vi "Splitter.vi"(6 "Selection Colors":T1={"Normal"=13816530, "Mouse-over"=0, "Selected"=9868950, "Selected Mouse-over"=9868950}, 7 "Settings UI Enqueuer":refnum<class "Message Enqueuer.lvclass">, 8 "Error In":errorcluster, 9 "Offset":T2, 10 "Scale Factor":dbl, 11 "Splitter Ref":refnum<vi>) -> (0 "Error Out":errorcluster, 3 "Splitter out":refnum<class "Splitter.lvclass">)   [LabVIEW 2017, in "Splitter.lvclass"]
uses:
  Splitter.lvclass
  D:/software/LabView_PaneRelief_2017/test/D/software/LabView_PaneRelief_2017/Classes/Panel Object/Panel Object.lvclass
  Typedefs/Point--Cluster.ctl
  <vilib>/ActorFramework/Message Enqueuer/Message Enqueuer.lvclass
  Typedefs/Selection Colors--Cluster.ctl
  Typedefs/Splitter Orientation--Enum.ctl
  Splitter.lvclass/Splitter.ctl
  Typedefs/Rectangle--Cluster.ctl
  Panel Object/Panel Object.lvclass/Panel Object.ctl
  Panel Object/Write Bounds.vi
  Panel Object/Write Settings UI Enqueuer.vi
  Panel Object/Write Selection Colors.vi
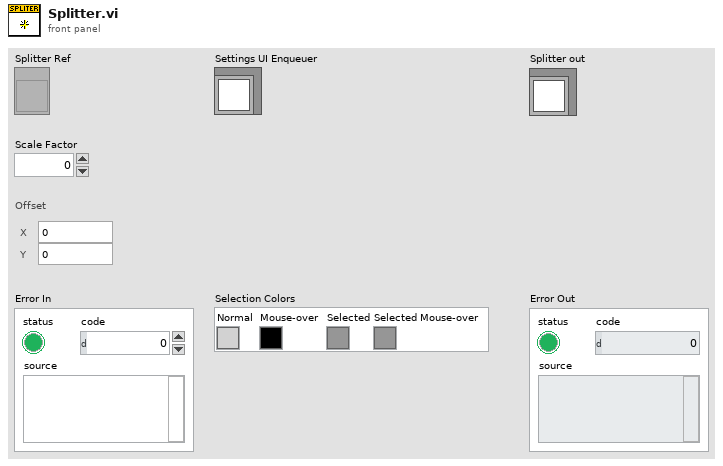
[diagram p1: front panel]
types:
  T1 = typedef "Selection Colors--Cluster.ctl" = cluster{"Normal":u32, "Mouse-over":u32, "Selected":u32, "Selected Mouse-over":u32}
  T2 = typedef "Point--Cluster.ctl" = cluster{"Horizontal":i32, "Vertical":i32}
  T3 = typedef "Splitter Orientation--Enum.ctl" = enum16{"Vertical", "Horizontal"}
  T4 = typedef "Rectangle--Cluster.ctl" = cluster{"X start":i32, "X end":i32, "Y start":i32, "Y end":i32}
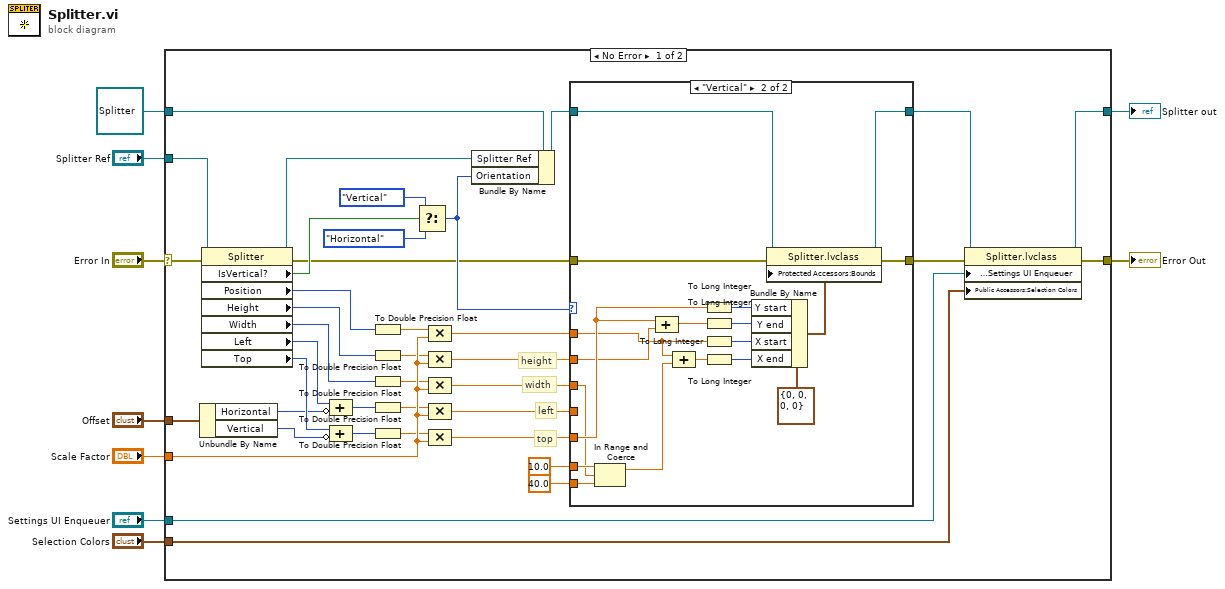
[diagram p0: block diagram]
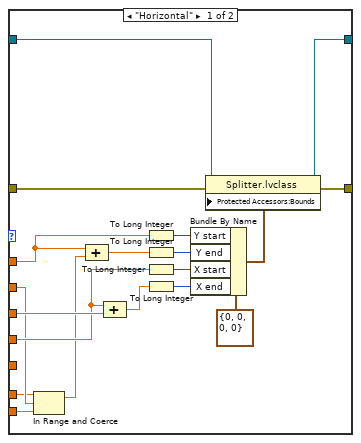
[diagram p2: hidden frame]
diagram:
  n1 = case shown="No Error" "Error In" {
    selector: "Error In" -> [w28 w88]
    tunnel: [w16 w88] -> w7
    tunnel: [w14 w87] -> w9
    tunnel: refnum<class "Splitter.lvclass"> refnum ("Splitter in") -> [w20 w87]
    tunnel: "Splitter Ref" -> [w26 _]
    tunnel: "Scale Factor" -> [w34 _]
    tunnel: "Offset" -> [w33 _]
    tunnel: "Settings UI Enqueuer" -> [w13 _]
    tunnel: "Selection Colors" -> [w12 _]
    frame No Error {
      # "top"
      # "left"
      # "width"
      # "height"
      n2 = Unbundle By Name(w33) -> ("Horizontal"=w35:i32, "Vertical"=w38:i32)
      n3 = property class="Splitter"(reference=w26, error in=w28) -> (reference out=w27:refnum<vi>, error out=w19:errorcluster, "IsVertical?"=w32:bool, "Position"=w48:i32, "Height"=w41:u32, "Width"=w44:u32, "Left"=w37:i32, "Top"=w39:i32)
      n4 = Compound Arithmetic op=ADD(w37, invert w35) -> (w36:i32)
      n5 = Compound Arithmetic op=ADD(w39, invert w38) -> (w40:i32)
      n6 = To Double Precision Float(number=w48) -> (double precision float=w25:dbl)
      n7 = To Double Precision Float(number=w41) -> (double precision float=w24:dbl)
      n8 = To Double Precision Float(number=w44) -> (double precision float=w23:dbl)
      n9 = To Double Precision Float(number=w36) -> (double precision float=w22:dbl)
      n10 = To Double Precision Float(number=w40) -> (double precision float=w21:dbl)
      n11 = Select(t=Splitter_Orientation--Enum."Vertical" ("Splitter Orientation"), s=w32, f=Splitter_Orientation--Enum."Horizontal" ("Splitter Orientation")) -> (s? t:f=w29:T3)
      n12 = Compound Arithmetic op=MULTIPLY(w25, w34) -> (w45:dbl)
      n13 = Compound Arithmetic op=MULTIPLY(w24, w34) -> (w46:dbl)
      n14 = Compound Arithmetic op=MULTIPLY(w23, w34) -> (w47:dbl)
      n15 = Compound Arithmetic op=MULTIPLY(w22, w34) -> (w43:dbl)
      n16 = Compound Arithmetic op=MULTIPLY(w21, w34) -> (w42:dbl)
      n17 = Bundle By Name(cluster=w20, "Splitter Ref"=w27, "Orientation"=w29) -> (w18:refnum<class "Splitter.lvclass">)
      n18 = case shown="\"Vertical\"" w29 {
        tunnel: w45 -> [w64 w83]
        tunnel: w43 -> [w66 _]
        tunnel: w46 -> [w52 w84]
        tunnel: w47 -> [w67 w70]
        tunnel: w42 -> [_ w85]
        tunnel: w19 -> [w58 w77]
        tunnel: [w57 w76] -> w17
        tunnel: [w56 w73] -> w15
        tunnel: w18 -> [w55 w74]
        tunnel: 10.0 ("upper limit") -> [w50 w72]
        tunnel: 40.0 ("upper limit") -> [w49 w71]
        frame "Horizontal" {
          # "Horizontal"
          n19 = In Range and Coerce(upper limit=w50, x=w52, lower limit=w49) -> (coerced(x)=w51:dbl)  [unwired: 1 out]
          n20 = Compound Arithmetic op=ADD(w64, w51) -> (w63:dbl)
          n21 = Compound Arithmetic op=ADD(w66, w67) -> (w65:dbl)
          n22 = To Long Integer(number=w64) -> (32bit integer=w62:i32)
          n23 = To Long Integer(number=w63) -> (32bit integer=w61:i32)
          n24 = To Long Integer(number=w66) -> (32bit integer=w60:i32)
          n25 = To Long Integer(number=w65) -> (32bit integer=w59:i32)
          n26 = Bundle By Name(cluster=T4 {"X start"=0, "X end"=0, "Y start"=0, "Y end"=0} ("Bounds"), "Y start"=w62, "Y end"=w61, "X start"=w60, "X end"=w59) -> (w53:T4)
          n27 = property class="Splitter.lvclass"(reference=w55, error in=w58, "Protected Accessors:Bounds"=w53) -> (reference out=w56:refnum<class "Splitter.lvclass">, error out=w57:errorcluster)
        }
        frame "Vertical" {
          # "Vertical"
          n28 = In Range and Coerce(upper limit=w72, x=w70, lower limit=w71) -> (coerced(x)=w69:dbl)  [unwired: 1 out]
          n29 = Compound Arithmetic op=ADD(w85, w84) -> (w86:dbl)
          n30 = Compound Arithmetic op=ADD(w83, w69) -> (w82:dbl)
          n31 = To Long Integer(number=w85) -> (32bit integer=w81:i32)
          n32 = To Long Integer(number=w86) -> (32bit integer=w80:i32)
          n33 = To Long Integer(number=w83) -> (32bit integer=w79:i32)
          n34 = To Long Integer(number=w82) -> (32bit integer=w78:i32)
          n35 = Bundle By Name(cluster=T4 {"X start"=0, "X end"=0, "Y start"=0, "Y end"=0} ("Bounds"), "Y start"=w81, "Y end"=w80, "X start"=w79, "X end"=w78) -> (w75:T4)
          n36 = property class="Splitter.lvclass"(reference=w74, error in=w77, "Protected Accessors:Bounds"=w75) -> (reference out=w73:refnum<class "Splitter.lvclass">, error out=w76:errorcluster)
        }
      }
      n37 = property class="Splitter.lvclass"(reference=w15, error in=w17, "Protected Accessors:Settings UI Enqueuer"=w13, "Public Accessors:Selection Colors"=w12) -> (reference out=w14:refnum<class "Splitter.lvclass">, error out=w16:errorcluster)
    }
    frame Error {
    }
  }
  "Splitter out" <- w9
  "Error Out" <- w7
